vi "SendReply.vi"(5 "ReplyQueue":refnum<queue>, 7 "CmdCtrl":T1, 9 "ReplyDataIn":variant, 10 "ASycnErrorIn":errorcluster, 11 "ErrorIn":errorcluster) -> (0 "ErrorOut":errorcluster)   [LabVIEW 2021, in "YActor.lvclass"]
uses:
  YActor.lvclass
  CmdCtrl.ctl
  AsyncErrorHandling.ctl
  CallMode.ctl
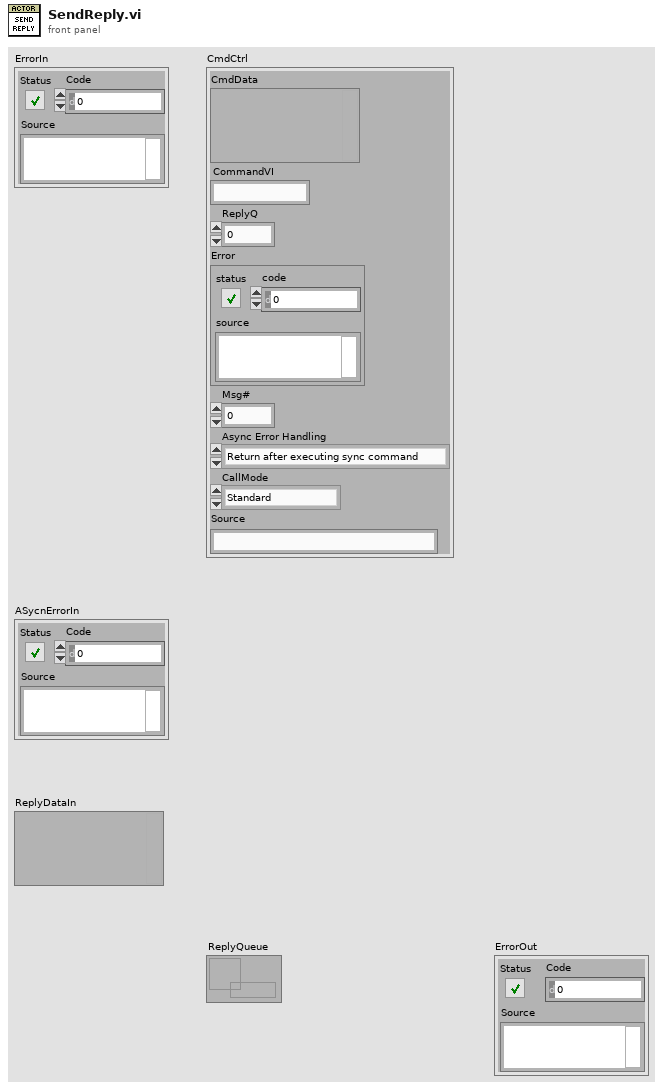
[diagram p1: front panel]
types:
  T1 = typedef "YActor.lvclass/CmdCtrl.ctl" = cluster{"CmdData":variant, "CommandVI":string, "ReplyQ":i64, "Error":errorcluster, "Msg#":u32, "Async Error Handling":T2, "CallMode":T3, "Source":string}
  T2 = typedef "YActor.lvclass/AsyncErrorHandling.ctl" = enum16{"Return after executing sync command", "Return before executing sync command", "Don't return error"}
  T3 = typedef "YActor.lvclass/CallMode.ctl" = enum16{"Standard", "Call&Collect"}
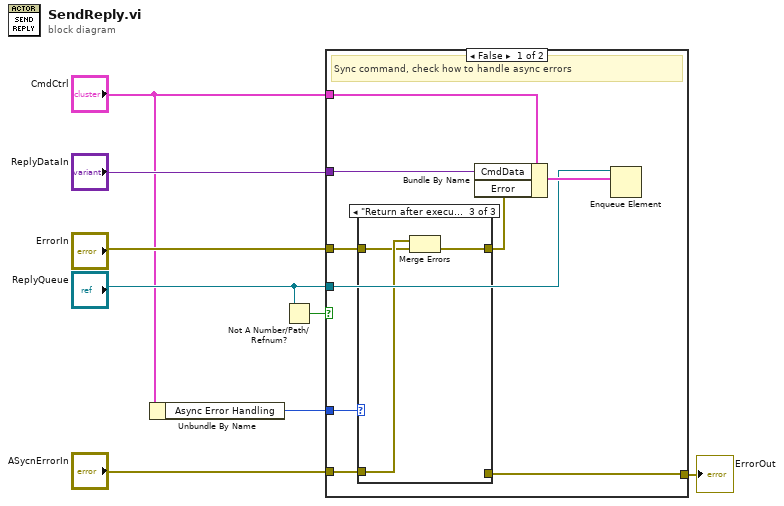
[diagram p0: block diagram]
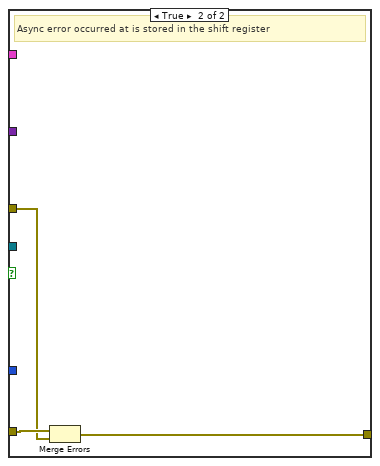
[diagram p4: hidden frame]
diagram:
  n1 = Unbundle By Name("CmdCtrl") -> ("Async Error Handling"=w2:T2)
  n2 = Not A Number/Path/Refnum?(number/path/refnum="ReplyQueue") -> (NaN/Path/Refnum?=w3:bool)
  n3 = case shown="False" w3 {
    tunnel: "ReplyDataIn" -> [w12 _]
    tunnel: "CmdCtrl" -> [w11 _]
    tunnel: "ReplyQueue" -> [w10 _]
    tunnel: "ErrorIn" -> [w17 w24]
    tunnel: "ASycnErrorIn" -> [w16 w25]
    tunnel: w2 -> [w9 _]
    tunnel: [w14 w23] -> w7
    frame False {
      # "Sync command, check how to handle async errors"
      n4 = case shown="\"Return after executing sync command\"" w9 {
        tunnel: w17 -> [w18 w19 w21]
        tunnel: w16 -> [_ _ w22]
        tunnel: [w18 _ w20] -> w15
        tunnel: [_ w19 _] -> w14
        frame "Return before executing sync command" {
        }
        frame "Don't return error" {
        }
        frame "Return after executing sync command" {
          n5 = Merge Errors(w22, w21) -> (w20:errorcluster)
        }
      }
      n6 = Bundle By Name(cluster=w11, "CmdData"=w12, "Error"=w15) -> (w13:T1)
      n7 = Enqueue Element(queue=w10, element=w13) -> ()  [unwired: 2 in, 3 out]
    }
    frame True {
      # "Async error occurred at is stored in the shift register"
      n8 = Merge Errors(w25, w24) -> (w23:errorcluster)
    }
  }
  "ErrorOut" <- w7
